vi "Reset.vi"(8 "error in (no error)":errorcluster, 11 "NI PXI Trigger in":refnum<class "NI PXI Trigger.lvclass">) -> (0 "error out":errorcluster, 3 "NI PXI Trigger out":refnum<class "NI PXI Trigger.lvclass">)   [LabVIEW 2020, in "NI DAQmx.lvlib" / "NI PXI Trigger.lvclass"]
uses:
  NI PXI Trigger.lvclass
  NI PXI Trigger.lvclass/NI PXI Trigger.ctl
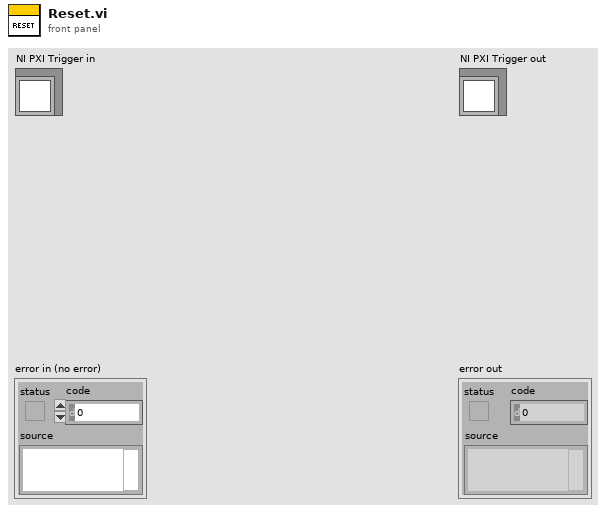
[diagram p1: front panel]
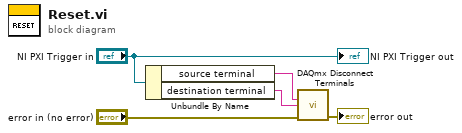
[diagram p0: block diagram]
diagram:
  n1 = Unbundle By Name("NI PXI Trigger in") -> ("source terminal"=w4:tag, "destination terminal"=w1:tag)
  n2 = call <vilib>:"DAQmx Disconnect Terminals.vi"("source terminal"=w4, "destination terminal"=w1, "error in"="error in (no error)") -> ("error out"=→"error out":errorcluster)  [unwired: 12 in]
  "NI PXI Trigger out" <- "NI PXI Trigger in"
